vi "FTP_TYPE.vi"(0 "connection ID":refnum<k5>, 1 "type (query)":enum16{"(query)", "ASCII", "binary"}(ring)=enum."binary", 2 "error in":errorcluster) -> (3 "connection ID out":refnum<k5>, 4 "reply string":string, 5 "Good Reply?":bool, 6 "error out":errorcluster)   [LabVIEW 2012]
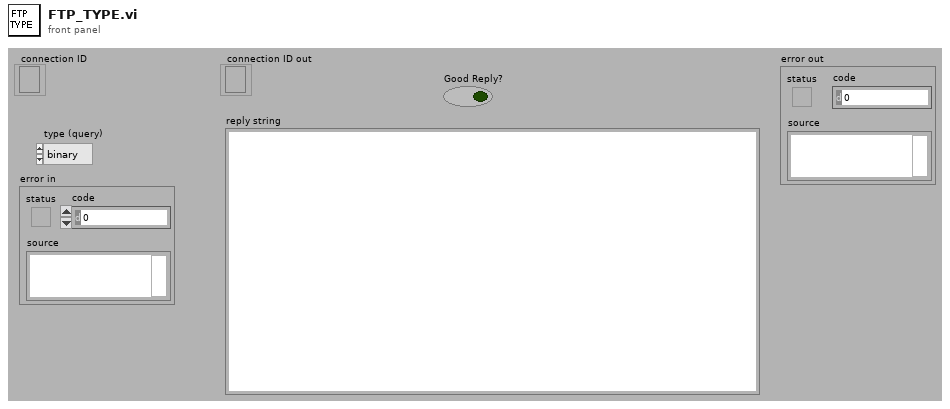
[diagram p1: front panel]
types:
  T1 = enum16{"unknown", "100 + Prelim", "200 + ", "300 + Intermed", "400 - Transient", "500 - Permanent"}
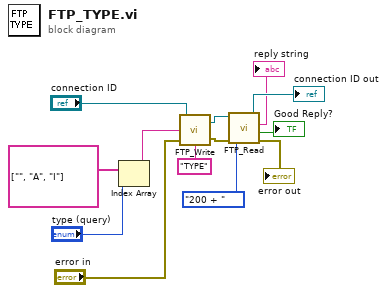
[diagram p0: block diagram]
diagram:
  n1 = Index Array(array=string[] ["", "A", "I"], index="type (query)") -> (element=w2:string)
  n2 = call <userlib>:"FTP_Write.vi"("Cmd"="TYPE", "error in"="error in", "data"=w2, "connection ID in"="connection ID") -> ("error out"=w6:errorcluster, "connection ID out"=w7:refnum<k5>)
  n3 = call <userlib>:"FTP_Read.vi"("error In"=w6, "expected class"=T1."200 + ", "connection ID"=w7) -> ("error out"=→"error out":errorcluster, "Good Reply?"=→"Good Reply?":bool, "reply string"=→"reply string":string, "connection ID out"=→"connection ID out":refnum<k5>)  [unwired: 1 out]
